vi "Teleop.vi"(10 "Match Info":T1={"Autonomous Elapsed Seconds"=0.0, "TeleOp Elapsed Seconds"=0.0, "Disabled Elapsed Seconds"=0.0, "Visited Autonomous"=FALSE, "Visited TeleOp"=FALSE, "Visited Disabled"=FALSE, "Autonomous Settings"={"Autonomous Style"=enum."Independent", "VI Refnum"=refnum}}, 11 "Call Context":T2) -> ()   [LabVIEW 2015]
doc: "This VI is called for each enabled TeleOp packet received from the DS. It is typically used to read from joysticks and other inputs and update I/O or setpoints for timed control loops. It should complete and return within 20 milliseconds or risk missing DS packets."
uses:
  <vilib>/Rock Robotics/WPI/DriverStation/WPI_DriverStationDerivedRobotMode.ctl
  <vilib>/Rock Robotics/WPI/DriverStation/WPI_DriverStationMatch Info.ctl
  Support Code/Logitech/F510/F510-X.vi
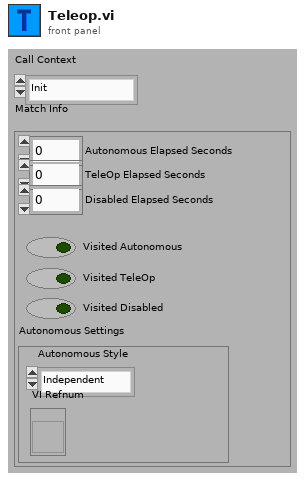
[diagram p1: front panel]
types:
  T1 = typedef "WPI_DriverStationMatch Info.ctl" = cluster{"Autonomous Elapsed Seconds":dbl, "TeleOp Elapsed Seconds":dbl, "Disabled Elapsed Seconds":dbl, "Visited Autonomous":bool, "Visited TeleOp":bool, "Visited Disabled":bool, "Autonomous Settings":cluster{"Autonomous Style":enum16{"Iterative", "Independent"}, "VI Refnum":refnum<vi>}}
  T2 = typedef "WPI_DriverStationDerivedRobotMode.ctl" = enum16{"Init", "Execute", "Stop"}
  T3 = cluster{"A":bool, "B":bool, "X":bool, "Y":bool, "LB":bool, "RB":bool, "Back":bool, "Start":bool, "LC":bool, "RC":bool, "LT":bool, "RT":bool}
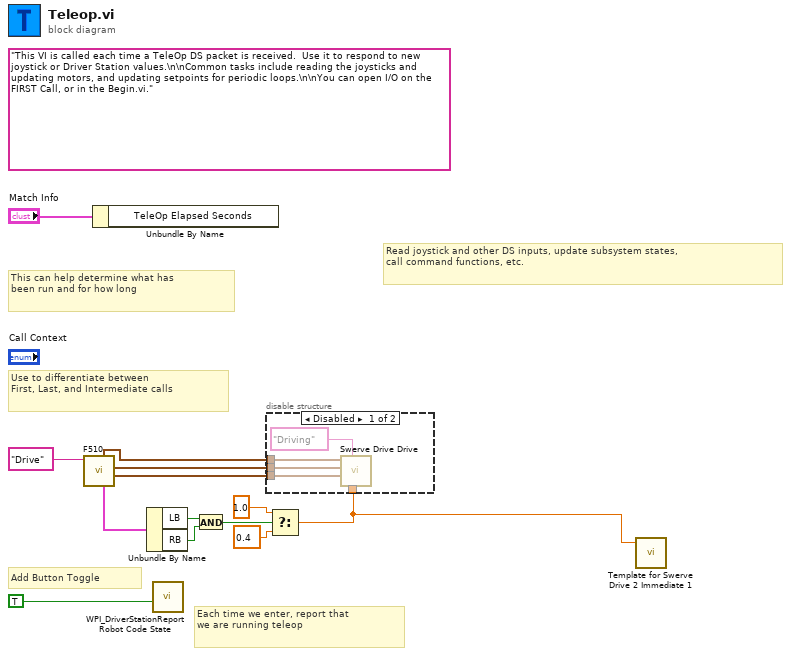
[diagram p0: block diagram]
diagram:
  (unwired) "This VI is called each time a TeleOp DS packet is received.  Use it to respond to new joystick or Driver Station values.\n\nCommon tasks include reading the joysticks and updating motors, and updating setpoints for periodic loops.\n\nYou can open I/O on the FIRST Call, or in the Begin.vi."
  # "Add Button Toggle"
  # "Read joystick and other DS inputs, update subsystem states,\ncall command functions, etc."
  # "Each time we enter, report that\nwe are running teleop"
  # "Use to differentiate between\nFirst, Last, and Intermediate calls"
  # "This can help determine what has\nbeen run and for how long"
  n1 = call-poly "F510.vi"("refnum name"="Drive") -> ("Right Stick"=w9:cluster{"X":dbl, "Y":dbl}, "Left Stick"=w10:cluster{"X":dbl, "Y":dbl}, "Buttons"=w7:T3, "Triggers"=w8:cluster{"Left":dbl, "Right":dbl})  [unwired: 4 in, 3 out]
  n2 = Unbundle By Name("Match Info") -> ()  [unwired: 1 out]
  n3 = Unbundle By Name(w7) -> ("LB"=w6:bool, "RB"=w5:bool)
  n4 = call <vilib>:"WPI_DriverStationReport Robot Code State.vi"("TeleOp"=TRUE ("Autonomous")) -> ()  [unwired: 10 in, 1 out]
  n5 = And(x=w6, y=w5) -> (x .and. y?=w4:bool)
  n6 = Select(t=1.0, s=w4, f=0.4) -> (s? t:f=w1:dbl)
  n7 = disable-structure shown="Disabled" {
    disable-tunnel: w10 -> [w17 _]
    disable-tunnel: w9 -> [w16 _]
    disable-tunnel: w8 -> [w15 _]
    disable-tunnel: w1 -> [w14 _]
    frame Disabled {
      n8 = call "Swerve Drive Drive.vi"("Speed Multiplier"=w14, "Description"="Driving", "Face Joystick Axes"=w16, "Strafe Joystick Axes"=w17, "Trigger Axes"=w15) -> ()  [unwired: 6 in, 1 out]
    }
    frame Enabled {
    }
  }
  n9 = call "Template for Swerve Drive 2 Immediate 1.vi"("Setpoint"=w1) -> ()  [unwired: 10 in, 1 out]
